vi "PAN_TCPSERVER_Close.vi"(8 "error in (no error)":errorcluster, 11 "listener ID":refnum<k5>) -> (0 "error out":errorcluster)   [LabVIEW 2016]
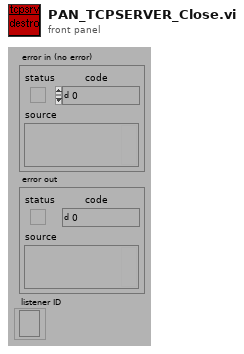
[diagram p1: front panel]
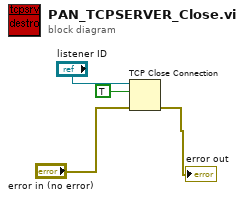
[diagram p0: block diagram]
diagram:
  n1 = TCP Close Connection(connection ID="listener ID", abort (F)=TRUE, error in (no error)="error in (no error)") -> (error out=→"error out":errorcluster)  [unwired: 1 out]
